vi "CoincidencePicture.vi"(4 "threshold":u32, 5 "Zoom":i32, 6 "new IMAGElsize":cluster{"x":u32, "Y":u32}, 7 "Image Pixels (U8)":u8[][](array[numeric]), 8 "Palette Number (gray)":T1(ring), 9 "Enum":T3(ring)) -> (0 "Palette Number (gray) 2":T1(ring), 1 "String":string, 3 "Image Out":T2)   [LabVIEW 2009]
uses:
  <vilib>/vision/Image Controls.llb/IMAQ Image.ctl
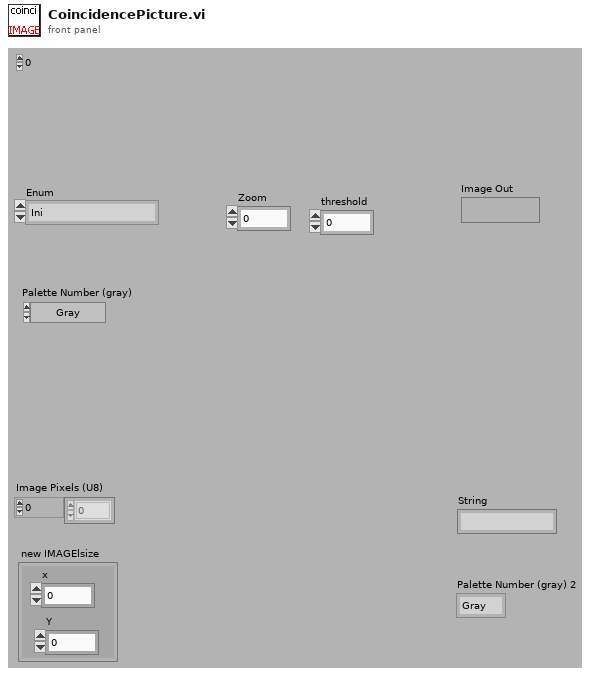
[diagram p1: front panel]
types:
  T1 = enum32{"Gray", "Binary", "Gradient", "Rainbow", "Temperature"}
  T2 = typedef "IMAQ Image.ctl" = refnum<image>
  T3 = enum16{"Ini", "Get", "Set", "Draw", "Colorpal", "Dump", "Zoom"}
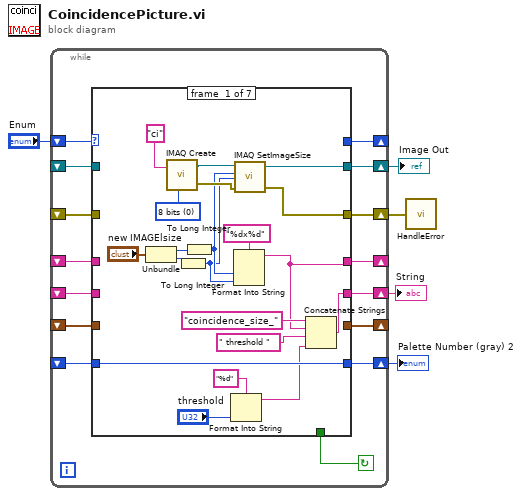
[diagram p0: block diagram]
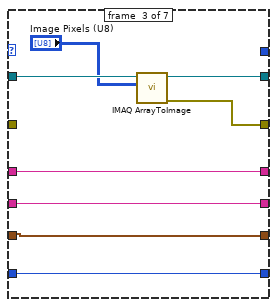
[diagram p3: hidden frame]
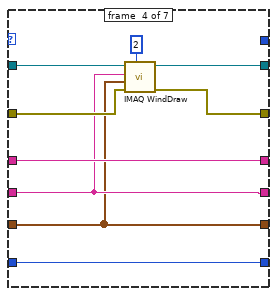
[diagram p4: hidden frame]
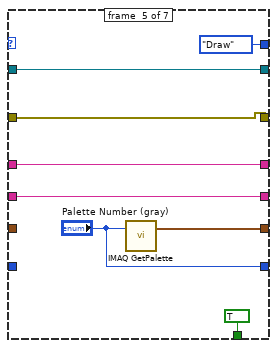
[diagram p5: hidden frame]
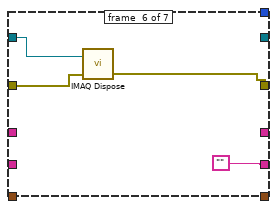
[diagram p6: hidden frame]
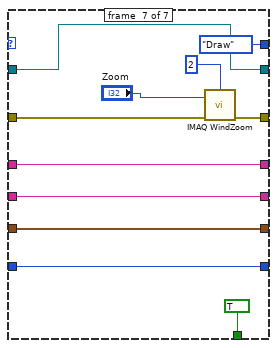
[diagram p7: hidden frame]
diagram:
  n1 = while {
    shift-right: [w20] -> w5
    shift-left: _ -> [w19]
    shift-right: [w18] -> w1
    shift-left: _ -> [w17]
    shift-right: [w15] -> _
    shift-left: "Enum" -> [w10]
    shift-right: [w14] -> _
    shift-left: _ -> [w13]
    shift-right: [w12] -> w3
    shift-left: _ -> [w11]
    shift-right: [w8] -> _
    shift-left: _ -> [w9]
    shift-right: [w7] -> w2
    shift-left: _ -> [w6]
    stop <- w16 continue-if-true
    n2 = case shown="\"Ini\", Default" w10 {
      tunnel: [w38 w46 w54 w62 w67 _ w81] -> w20
      tunnel: w19 -> [_ w46 w53 w63 w67 w75 w81]
      tunnel: [w36 w45 w51 w61 w68 w73 w84] -> w18
      tunnel: w17 -> [_ w45 _ w60 w68 w74 w85]
      tunnel: [_ _ _ _ TRUE _ TRUE] -> w16
      tunnel: [_ _ _ _ T3."Draw" ("Enum") _ T3."Draw" ("Enum")] -> w15
      tunnel: [w30 w44 w50 w57 w69 _ w77] -> w14
      tunnel: w13 -> [_ w44 w50 w57 w69 _ w77]
      tunnel: [w29 w43 w49 w56 w70 "" w83] -> w12
      tunnel: w11 -> [_ w43 w49 w56 w70 _ w83]
      tunnel: w9 -> [_ w42 w48 w55 _ _ w78]
      tunnel: [_ w42 w48 w55 w71 _ w78] -> w8
      tunnel: [w28 w41 w47 w58 "Palette Number (gray)" _ w76] -> w7
      tunnel: w6 -> [w28 w41 w47 w58 _ _ w76]
      frame #0 {
        w37 = u32 0 items=["8 bits", "16 bits", "Float", "Complex", "RGB", "HSL"] ("Image Type")
        n3 = Unbundle("new IMAGElsize") -> ("x"=w22:u32, "Y"=w21:u32)
        n4 = call "IMAQ Create"("Image Name"="ci", "Image Type"=w37) -> ("New Image"=w39:T2, "error out"=w40:errorcluster)  [unwired: 3 in]
        n5 = To Long Integer(number=w21) -> (32bit integer=w32:i32)
        n6 = To Long Integer(number=w22) -> (32bit integer=w33:i32)
        n7 = Format Into String(format string="%d", "threshold") -> (resulting string=w26:string)  [unwired: 2 in, 1 out]
        n8 = Format Into String(format string="%dx%d", w33, w32) -> (resulting string=w30:string)  [unwired: 2 in, 1 out]
        n9 = call "IMAQ SetImageSize"("error in (no error)"=w40, "Y Resolution"=w32, "X Resolution"=w33, "Image"=w39) -> ("error out"=w36:errorcluster, "Image Out"=w38:T2)  [unwired: 1 in]
        n10 = Concatenate Strings("coincidence_size_" ("Title"), w30, " threshold " ("string"), w26) -> (w29:string)
      }
      frame #1 {
      }
      frame #2 {
        n11 = call "IMAQ ArrayToImage"("Image Pixels (U8)"="Image Pixels (U8)", "Image"=w53) -> ("error out"=w51:errorcluster, "Image Out"=w54:T2)  [unwired: 8 in]
      }
      frame #3 {
        n12 = call "IMAQ WindDraw"("Window Number (0...15)"=2, "error in (no error)"=w60, "Color Palette"=w55, "Title"=w56, "Image"=w63) -> ("error out"=w61:errorcluster, "Image Out (duplicate)"=w62:T2)  [unwired: 5 in]
      }
      frame #4 {
        n13 = call "IMAQ GetPalette"("Palette Number (gray)"="Palette Number (gray)") -> ("Color Palette"=w71:cluster{"Red":u8, "Green":u8, "Blue":u8}[])  [unwired: 4 in, 1 out]
      }
      frame #5 {
        n14 = call "IMAQ Dispose"("Image"=w75, "error in (no error)"=w74) -> ("error out"=w73:errorcluster)  [unwired: 4 in]
      }
      frame #6 {
        n15 = call "IMAQ WindZoom"("error in (no error)"=w85, "Zoom Factor"="Zoom", "Window Number (0...15)"=2) -> ("error out"=w84:errorcluster)  [unwired: 3 in, 2 out]
      }
    }
  }
  "Image Out" <- w5
  "String" <- w3
  "Palette Number (gray) 2" <- w2
  n16 = call "HandleError.vi"("error in (no error)"=w1) -> ()
